vi "Receive notification.vi"(8 "error in":errorcluster, 10 "Variant":variant, 11 "notifier in":refnum<notifier>) -> (0 "error out":errorcluster, 1 "message":string, 2 "data":variant, 3 "notifier out":refnum<notifier>)   [LabVIEW 2020]
uses:
  _controls/Notifier Cluster.ctl
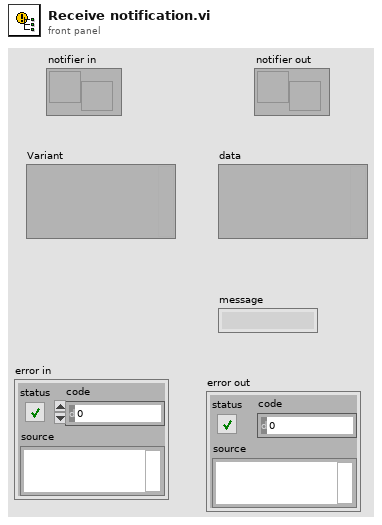
[diagram p1: front panel]
types:
  T1 = typedef "Notifier Cluster.ctl" = cluster{"message":string, "data":variant}
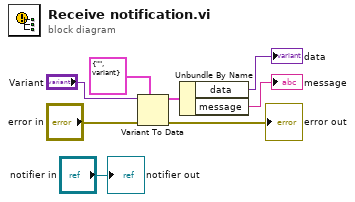
[diagram p0: block diagram]
diagram:
  n1 = Variant To Data(error in="error in", type=T1 {"message"="", "data"=variant}, Variant="Variant") -> (data=w5:T1, error out=→"error out":errorcluster)
  n2 = Unbundle By Name(w5) -> ("data"=→"data":variant, "message"=→"message":string)
  "notifier out" <- "notifier in"
